vi "WPC stats scrape.vi"() -> (2 "redacted?":bool, 3 "WPC Player Stats":T1[](array[typedef]) {"Date Updated" format="%<%m/%d/%Y>T"})   [LabVIEW 2021]
uses:
  WPC Player and Financial Stats.ctl
  <vilib>/httpClient/LabVIEWHTTPClient.lvlib
panel:
  out "body":string
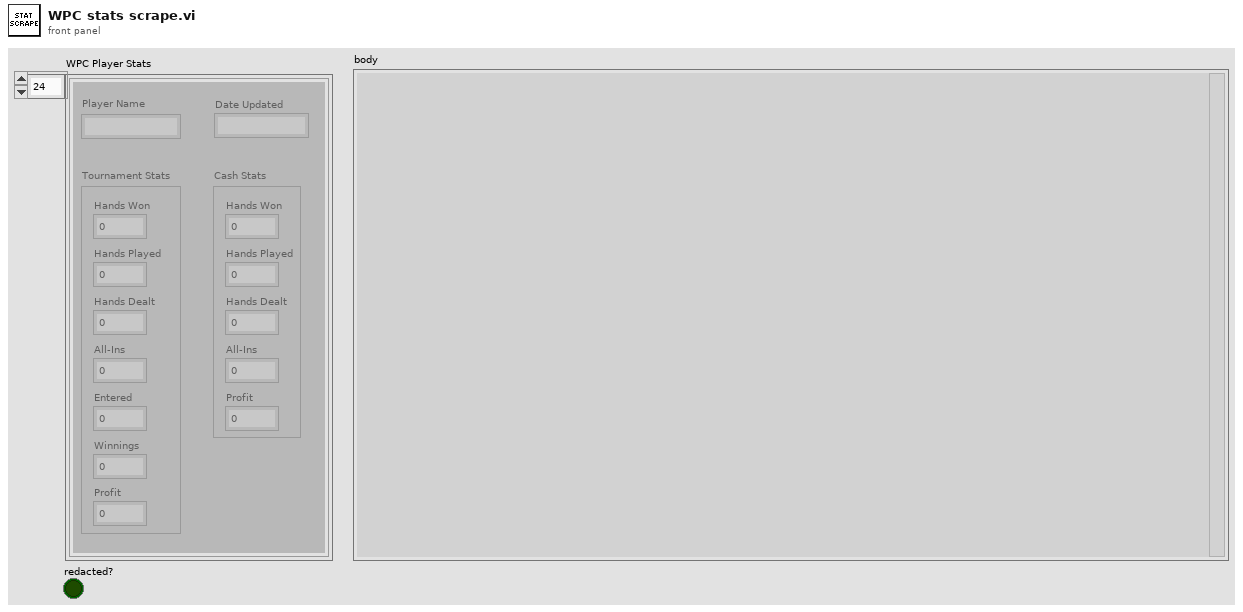
[diagram p1: front panel]
types:
  T1 = typedef "WPC Player and Financial Stats.ctl" = cluster{"Player Name":string, "Date Updated":timestamp, "Tournament Stats":cluster{"Hands Won":i32, "Hands Played":i32, "Hands Dealt":i32, "All-Ins":i32, "Entered":i32, "Winnings":dbl, "Profit":dbl}, "Cash Stats":cluster{"Hands Won":i32, "Hands Played":i32, "Hands Dealt":i32, "All-Ins":i32, "Profit":dbl}}
  T2 = cluster{"Player":string, "Tournament Winings":dbl, "Tournament Profit":dbl, "Cashes":dbl}[]
  T3 = cluster{"Hands Won":u32, "Hands Played":u32, "Hands Dealt":u32, "All-Ins":u32}[]
  T4 = cluster{"Hands Won":u32, "Hands Played":u32, "Hands Dealt":u32, "All-Ins":u32, "Entered":u32}[]
  T5 = cluster{"[0]":dbl, "[1]":dbl, "[2]":dbl, "[3]":dbl, "[4]":dbl, "[5]":dbl, "[6]":dbl}
  T6 = cluster{"[0]":dbl, "[1]":dbl, "[2]":dbl, "[3]":dbl, "[4]":dbl}
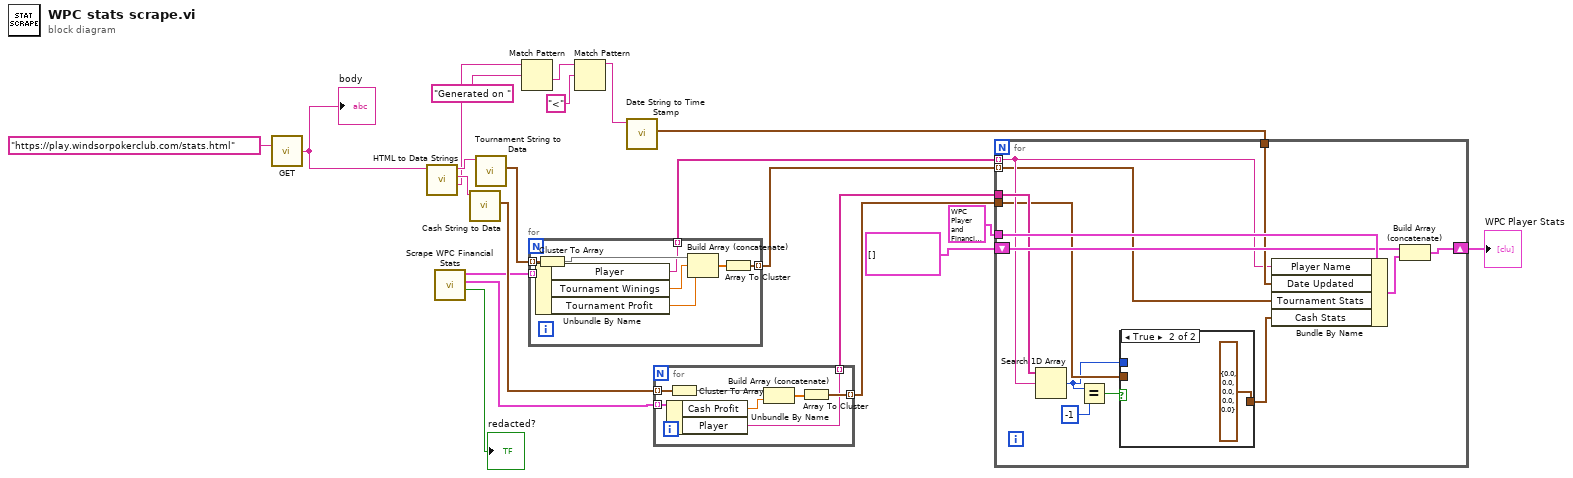
[diagram p0: block diagram]
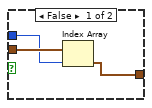
[diagram p2: hidden frame]
diagram:
  n1 = call <vilib>:"GET.vi"("url"="https://play.windsorpokerclub.com/stats.html") -> ("body"=w11:string)  [unwired: 11 in, 3 out]
  "body" <- w11
  n2 = call "HTML to Data Strings.vi"("input string"=w11) -> ("output string"=w10:string, "Cash Data String"=w20:string, "Tournament Data String"=w19:string)  [unwired: 8 in]
  n3 = call "Scrape WPC Financial Stats.vi"() -> ("redacted?"=→"redacted?":bool, "WPC Financial Cash Stats"=w3:cluster{"Player":string, "Cash Profit":dbl}[], "WPC Financial Tournament Stats"=w4:T2)  [unwired: 8 in, 1 out]
  n4 = call "Cash String to Data.vi"("Cash Data String"=w20) -> ("Cash Data Array"=w5:T3)  [unwired: 9 in, 1 out]
  n5 = call "Tournament String to Data.vi"("Tournament Data String"=w19) -> ("Tournament Data Array"=w6:T4)  [unwired: 9 in, 1 out]
  n6 = Match Pattern(string=w10, regular expression="Generated on ") -> (after substring=w13:string)  [unwired: 1 in, 3 out]
  n7 = for {
    tunnel: w6 -> [w30] mode=indexing
    tunnel: w4 -> [w29] mode=indexing
    tunnel: [w24] -> w18 mode=indexing
    tunnel: [w23] -> w2 mode=indexing
    n8 = Unbundle By Name(w29) -> ("Player"=w23:string, "Tournament Winings"=w27:dbl, "Tournament Profit"=w26:dbl)
    n9 = Cluster To Array(cluster=w30) -> (array=w28:u32[])
    n10 = Build Array (concatenate)(w28, w27, w26) -> (w25:dbl[])
    n11 = Array To Cluster(array=w25) -> (cluster=w24:T5)
  }
  n12 = Match Pattern(string=w13, regular expression="<") -> (before substring=w8:string)  [unwired: 1 in, 3 out]
  n13 = call "Date String to Time Stamp.vi"("Date String"=w8) -> ("Time Stamp"=w21:timestamp)  [unwired: 10 in]
  n14 = for {
    tunnel: w5 -> [w37] mode=indexing
    tunnel: w3 -> [w36] mode=indexing
    tunnel: [w32] -> w17 mode=indexing
    tunnel: [w31] -> w1 mode=indexing
    n15 = Unbundle By Name(w36) -> ("Cash Profit"=w34:dbl, "Player"=w31:string)
    n16 = Cluster To Array(cluster=w37) -> (array=w35:u32[])
    n17 = Build Array (concatenate)(w35, w34) -> (w33:dbl[])
    n18 = Array To Cluster(array=w33) -> (cluster=w32:T6)
  }
  n19 = for {
    shift-right: [w49] -> w14
    shift-left: T1[] [] ("WPC Player Stats") -> [w48]
    tunnel: T1 {"Player Name"="", "Date Updated"=timestamp(0 s since 1904-01-01), "Tournament Stats"={"Hands Won"=0, "Hands Played"=0, "Hands Dealt"=0, "All-Ins"=0, "Entered"=0, "Winnings"=0.0, "Profit"=0.0}, "Cash Stats"={"Hands Won"=0, "Hands Played"=0, "Hands Dealt"=0, "All-Ins"=0, "Profit"=0.0}} ("WPC Player Stats") -> [w50]
    tunnel: w21 -> [w47]
    tunnel: w2 -> [w45] mode=indexing
    tunnel: w18 -> [w39] mode=indexing
    tunnel: w1 -> [w46]
    tunnel: w17 -> [w42]
    n20 = Search 1D Array(1D array=w46, element=w45) -> (index of element=w41:i32)  [unwired: 1 in]
    n21 = Equal?(x=w41, y=-1) -> (x = y?=w43:bool)
    n22 = case shown="True" w43 {
      tunnel: [w51 T6 {"[0]"=0.0, "[1]"=0.0, "[2]"=0.0, "[3]"=0.0, "[4]"=0.0}] -> w38
      tunnel: w42 -> [w53 _]
      tunnel: w41 -> [w52 _]
      frame False {
        n23 = Index Array(array=w53, index=w52) -> (element=w51:T6)
      }
      frame True {
      }
    }
    n24 = Bundle By Name(cluster=w50, "Player Name"=w45, "Date Updated"=w47, "Tournament Stats"=w39, "Cash Stats"=w38) -> (w40:T1)
    n25 = Build Array (concatenate)(w48, w40) -> (w49:T1[])
  }
  "WPC Player Stats" <- w14
